vi "Change Flame Level.vi"(9 "Increment?":bool, 11 "Boiler Data":T1) -> (1 "Time Increment":u32, 2 "Limit?":bool, 3 "Flame Level":u32)   [LabVIEW 2022 SP3, in "Boiler.lvlib"]
doc: "Increment or decrement the flame level of the boiler."
uses:
  Boiler.lvlib
  Boiler Data.ctl
  Boiler UI Data.ctl
  Boiler Configuration.ctl
  Boiler References.ctl
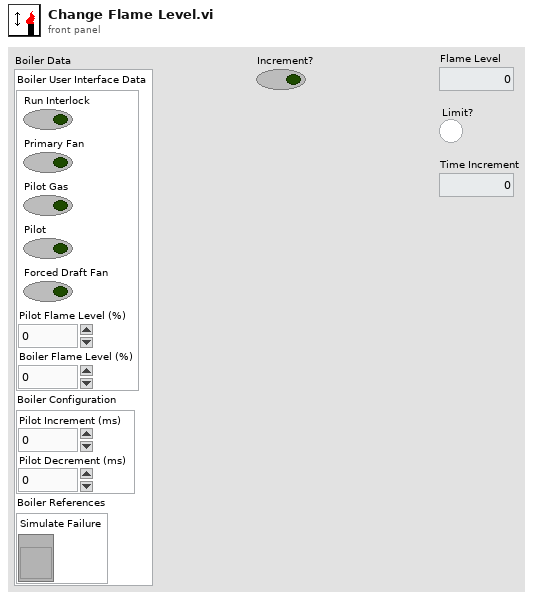
[diagram p1: front panel]
types:
  T1 = typedef "Boiler.lvlib/Boiler Data.ctl" = cluster{"Boiler User Interface Data":T2, "Boiler Configuration":T3, "Boiler References":T4}
  T2 = typedef "Boiler.lvlib/Boiler UI Data.ctl" = cluster{"Run Interlock":bool, "Primary Fan":bool, "Pilot Gas":bool, "Pilot":bool, "Forced Draft Fan":bool, "Pilot Flame Level (%)":u32, "Boiler Flame Level (%)":u32}
  T3 = typedef "Boiler.lvlib/Boiler Configuration.ctl" = cluster{"Pilot Increment (ms)":u32, "Pilot Decrement (ms)":u32}
  T4 = typedef "Boiler.lvlib/Boiler References.ctl" = cluster{"Simulate Failure":refnum<vi>}
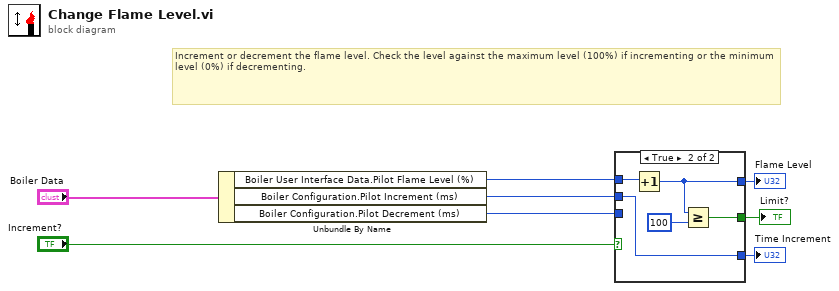
[diagram p0: block diagram]
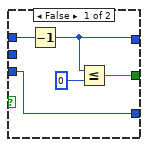
[diagram p2: hidden frame]
diagram:
  # "Increment or decrement the flame level. Check the level against the maximum level (100%) if incrementing or the minimum level (0%) if decrementing."
  n1 = Unbundle By Name("Boiler Data") -> ("Boiler User Interface Data.Pilot Flame Level (%)"=w3:u32, "Boiler Configuration.Pilot Increment (ms)"=w7:u32, "Boiler Configuration.Pilot Decrement (ms)"=w8:u32)
  n2 = case shown="True" "Increment?" {
    tunnel: w3 -> [w13 w18]
    tunnel: [w10 w17] -> w2
    tunnel: [w11 w15] -> w5
    tunnel: [w9 w14] -> w1
    tunnel: w7 -> [_ w14]
    tunnel: w8 -> [w9 _]
    frame False {
      n3 = Decrement(x=w13) -> (x-1=w10:u32)
      n4 = Less Or Equal?(x=w10, y=u32 0) -> (x <= y?=w11:bool)
    }
    frame True {
      n5 = Increment(x=w18) -> (x+1=w17:u32)
      n6 = Greater Or Equal?(x=w17, y=u32 100) -> (x >= y?=w15:bool)
    }
  }
  "Limit?" <- w5
  "Flame Level" <- w2
  "Time Increment" <- w1
